vi "restar inventario.vi"(10 "String":string, 11 "Productos":T1(array[cluster])) -> (3 "Array":T1(array[cluster]))   [LabVIEW 2020, in "Productos.lvlib"]
uses:
  Productos.lvlib
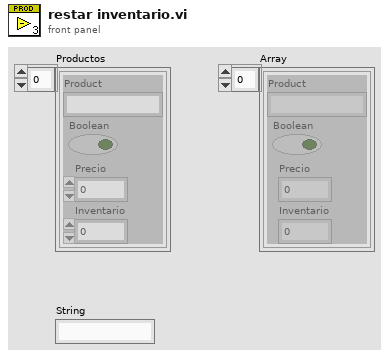
[diagram p1: front panel]
types:
  T1 = cluster{"Product":string, "Boolean":bool, "Precio":dbl, "Inventario":dbl}[]
  T2 = cluster{"Product":string, "Boolean":bool, "Precio":dbl, "Inventario":dbl}
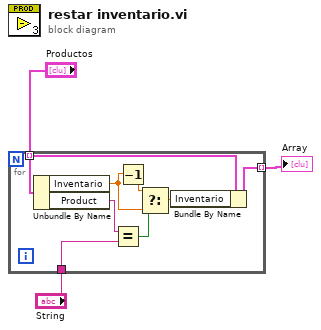
[diagram p0: block diagram]
diagram:
  n1 = for {
    tunnel: "Productos" -> [w10] mode=indexing
    tunnel: [w11] -> w3 mode=indexing
    tunnel: "String" -> [w8]
    n2 = Unbundle By Name(w10) -> ("Inventario"=w5:dbl, "Product"=w9:string)
    n3 = Equal?(x=w9, y=w8) -> (x = y?=w7:bool)
    n4 = Decrement(x=w5) -> (x-1=w4:dbl)
    n5 = Select(t=w4, s=w7, f=w5) -> (s? t:f=w6:dbl)
    n6 = Bundle By Name(cluster=w10, "Inventario"=w6) -> (w11:T2)
  }
  "Array" <- w3
